vi "Test Diagram Get Constants.vi"() -> ()   [LabVIEW 2014]
panel:
  out "Array 3":string[](array[string])
  out "alltop objects refs[]":string[](array[string])
  out "Array 2":i32[](array[numeric])
  out "Array":string[](array[string])
  in  "error in":errorcluster
  in  "VI path":path=path "C:/Users/lubo/Documents/LabView/LabVIEW-Universal-Transcriptor/Test/Examples For Parsing/Example Diagram Constants.vi"
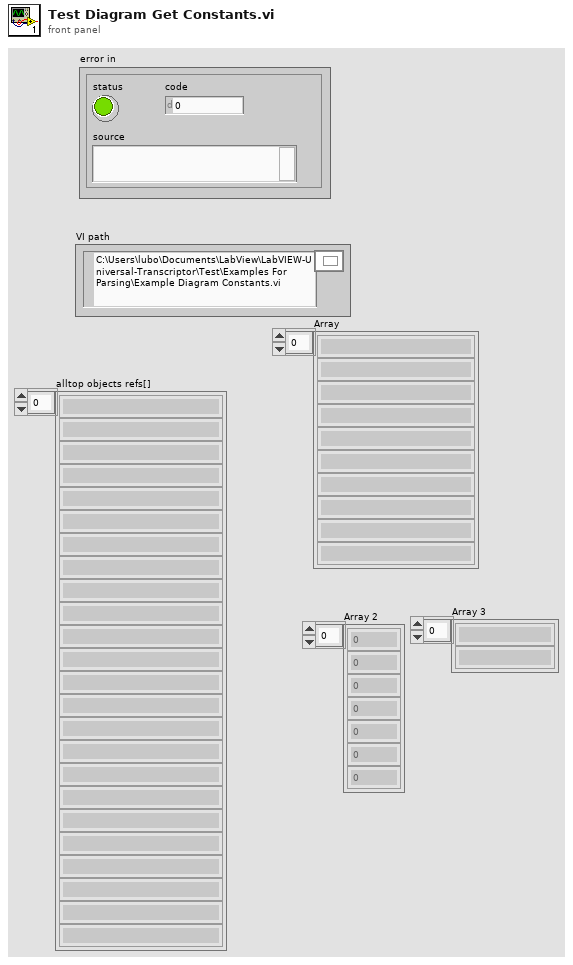
[diagram p1: front panel]
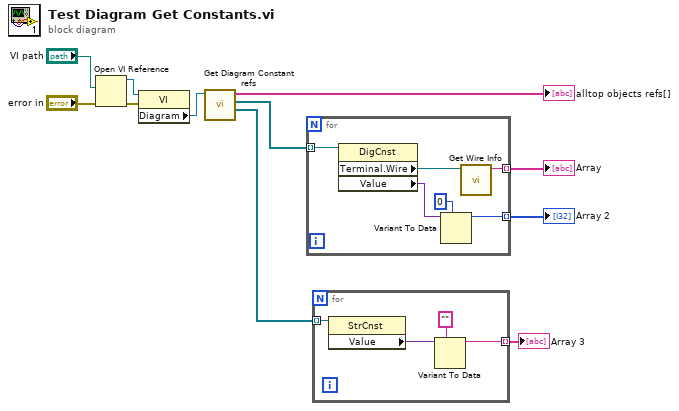
[diagram p0: block diagram]
diagram:
  n1 = Open VI Reference(vi path="VI path", error in (no error)="error in") -> (vi reference=w8:refnum<vi>, error out=w9:errorcluster)  [unwired: 4 in]
  n2 = property on="Property Node" class="VI"(reference=w8, error in=w9) -> ("Diagram"=w7:refnum<vi>)  [unwired: 2 out]
  n3 = call "Get Diagram Constant refs.vi"("Diagram ref."=w7) -> ("StringConstant refs[]"=w2:refnum<vi>[], "DigitalNumericConstant refs[]"=w6:refnum<vi>[], "alltop objects refs[]"=→"alltop objects refs[]":string[])  [unwired: 8 in]
  n4 = for {
    tunnel: w6 -> [w17] mode=indexing
    tunnel: [w15] -> w5 mode=indexing
    tunnel: [w12] -> w4 mode=indexing
    n5 = property class="DigCnst"(reference=w17) -> ("Terminal.Wire"=w16:refnum<vi>, "Value"=w14:variant)  [unwired: 1 in, 2 out]
    n6 = Variant To Data(type=0, Variant=w14) -> (data=w12:i32)  [unwired: 1 in, 1 out]
    n7 = call "Get Wire Info.vi"("Wire"=w16) -> ("wire label"=w15:string)  [unwired: 9 in, 1 out]
  }
  "Array" <- w5
  "Array 2" <- w4
  n8 = for {
    tunnel: w2 -> [w21] mode=indexing
    tunnel: [w18] -> w1 mode=indexing
    n9 = property class="StrCnst"(reference=w21) -> ("Value"=w20:variant)  [unwired: 1 in, 2 out]
    n10 = Variant To Data(type="", Variant=w20) -> (data=w18:string)  [unwired: 1 in, 1 out]
  }
  "Array 3" <- w1
